vi "Ramping.vi"(0 "Process Variable":dbl, 5 "First Ramp Point":dbl, 7 "First Ramp Speed":dbl, 9 "Second Ramp Point":dbl, 11 "Second Ramp Speed":dbl) -> (8 "Output Power":dbl)   [LabVIEW 2014]
panel:
  in  "Direction (T=UP)":bool
  in  "Initial Speed":dbl
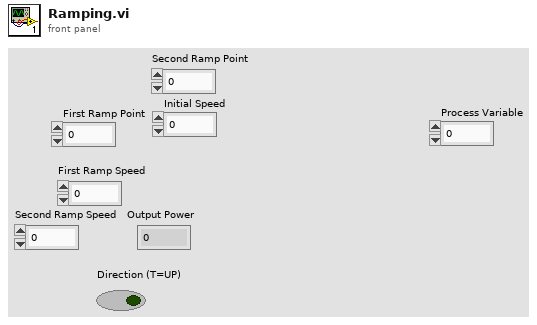
[diagram p1: front panel]
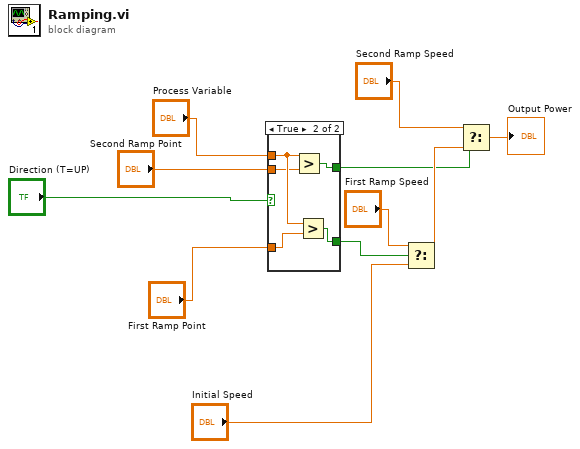
[diagram p0: block diagram]
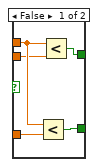
[diagram p2: hidden frame]
diagram:
  n1 = case shown="True" "Direction (T=UP)" {
    tunnel: [w15 w21] -> w8
    tunnel: [w16 w20] -> w7
    tunnel: "Process Variable" -> [w14 w19]
    tunnel: "First Ramp Point" -> [w13 w17]
    tunnel: "Second Ramp Point" -> [w12 w18]
    frame False {
      n2 = Less?(x=w14, y=w13) -> (x < y?=w16:bool)
      n3 = Less?(x=w14, y=w12) -> (x < y?=w15:bool)
    }
    frame True {
      n4 = Greater?(x=w19, y=w18) -> (0:w21:bool)
      n5 = Greater?(x=w19, y=w17) -> (0:w20:bool)
    }
  }
  n6 = Select(t="First Ramp Speed", s=w7, f="Initial Speed") -> (s? t:f=w11:dbl)
  n7 = Select(t="Second Ramp Speed", s=w8, f=w11) -> (s? t:f=→"Output Power":dbl)
